vi "Mavlink Message Decode.vi"(0 "VISA in":refnum<visa-resource-name>, 1 "mav_msg":T15, 3 "error_in":errorcluster) -> (7 "VISA out":refnum<visa-resource-name>, 10 "error_out":errorcluster)   [LabVIEW 2023]
panel:
  out "AUTOPILOT_VERSION":T1
  out "VIBRATION":T2
  out "AOA_SSA":cluster{"time_usec":u64, "AOA":sgl, "SSA":sgl}
  out "AHRS3":T3
  out "AHRS":T4
  out "TERRAIN_REPORT":T5
  out "HEARTBEAT":T6
  out "POWER_STATUS":T7
  out "TIMESYNC":T8
  out "STATUSTEXT":T9(array[cluster])
  out "POSITION_TARGET_GLOBAL_INT":T10
  out "PARAM_VALUE":T11
  out "VFR_HUD":T12
  out "RC_CHANNELS":T13
  out "MISSION_CURRENT":T14
  out "NAV_CONTROLLER_OUTPUT":T16
  out "SERVO_OUTPUT_RAW":T17
  out "GLOBAL_POSITION_INT":T18
  out "ATTITUDE":T19
  out "SCALED_PRESSURE":T20
  out "RAW_IMU":T21
  out "GPS_RAW_INT":T22
  out "SYSTEM_TIME":T23
  out "SYS_STATUS":T24
  out "Message":u32[](array[numeric])
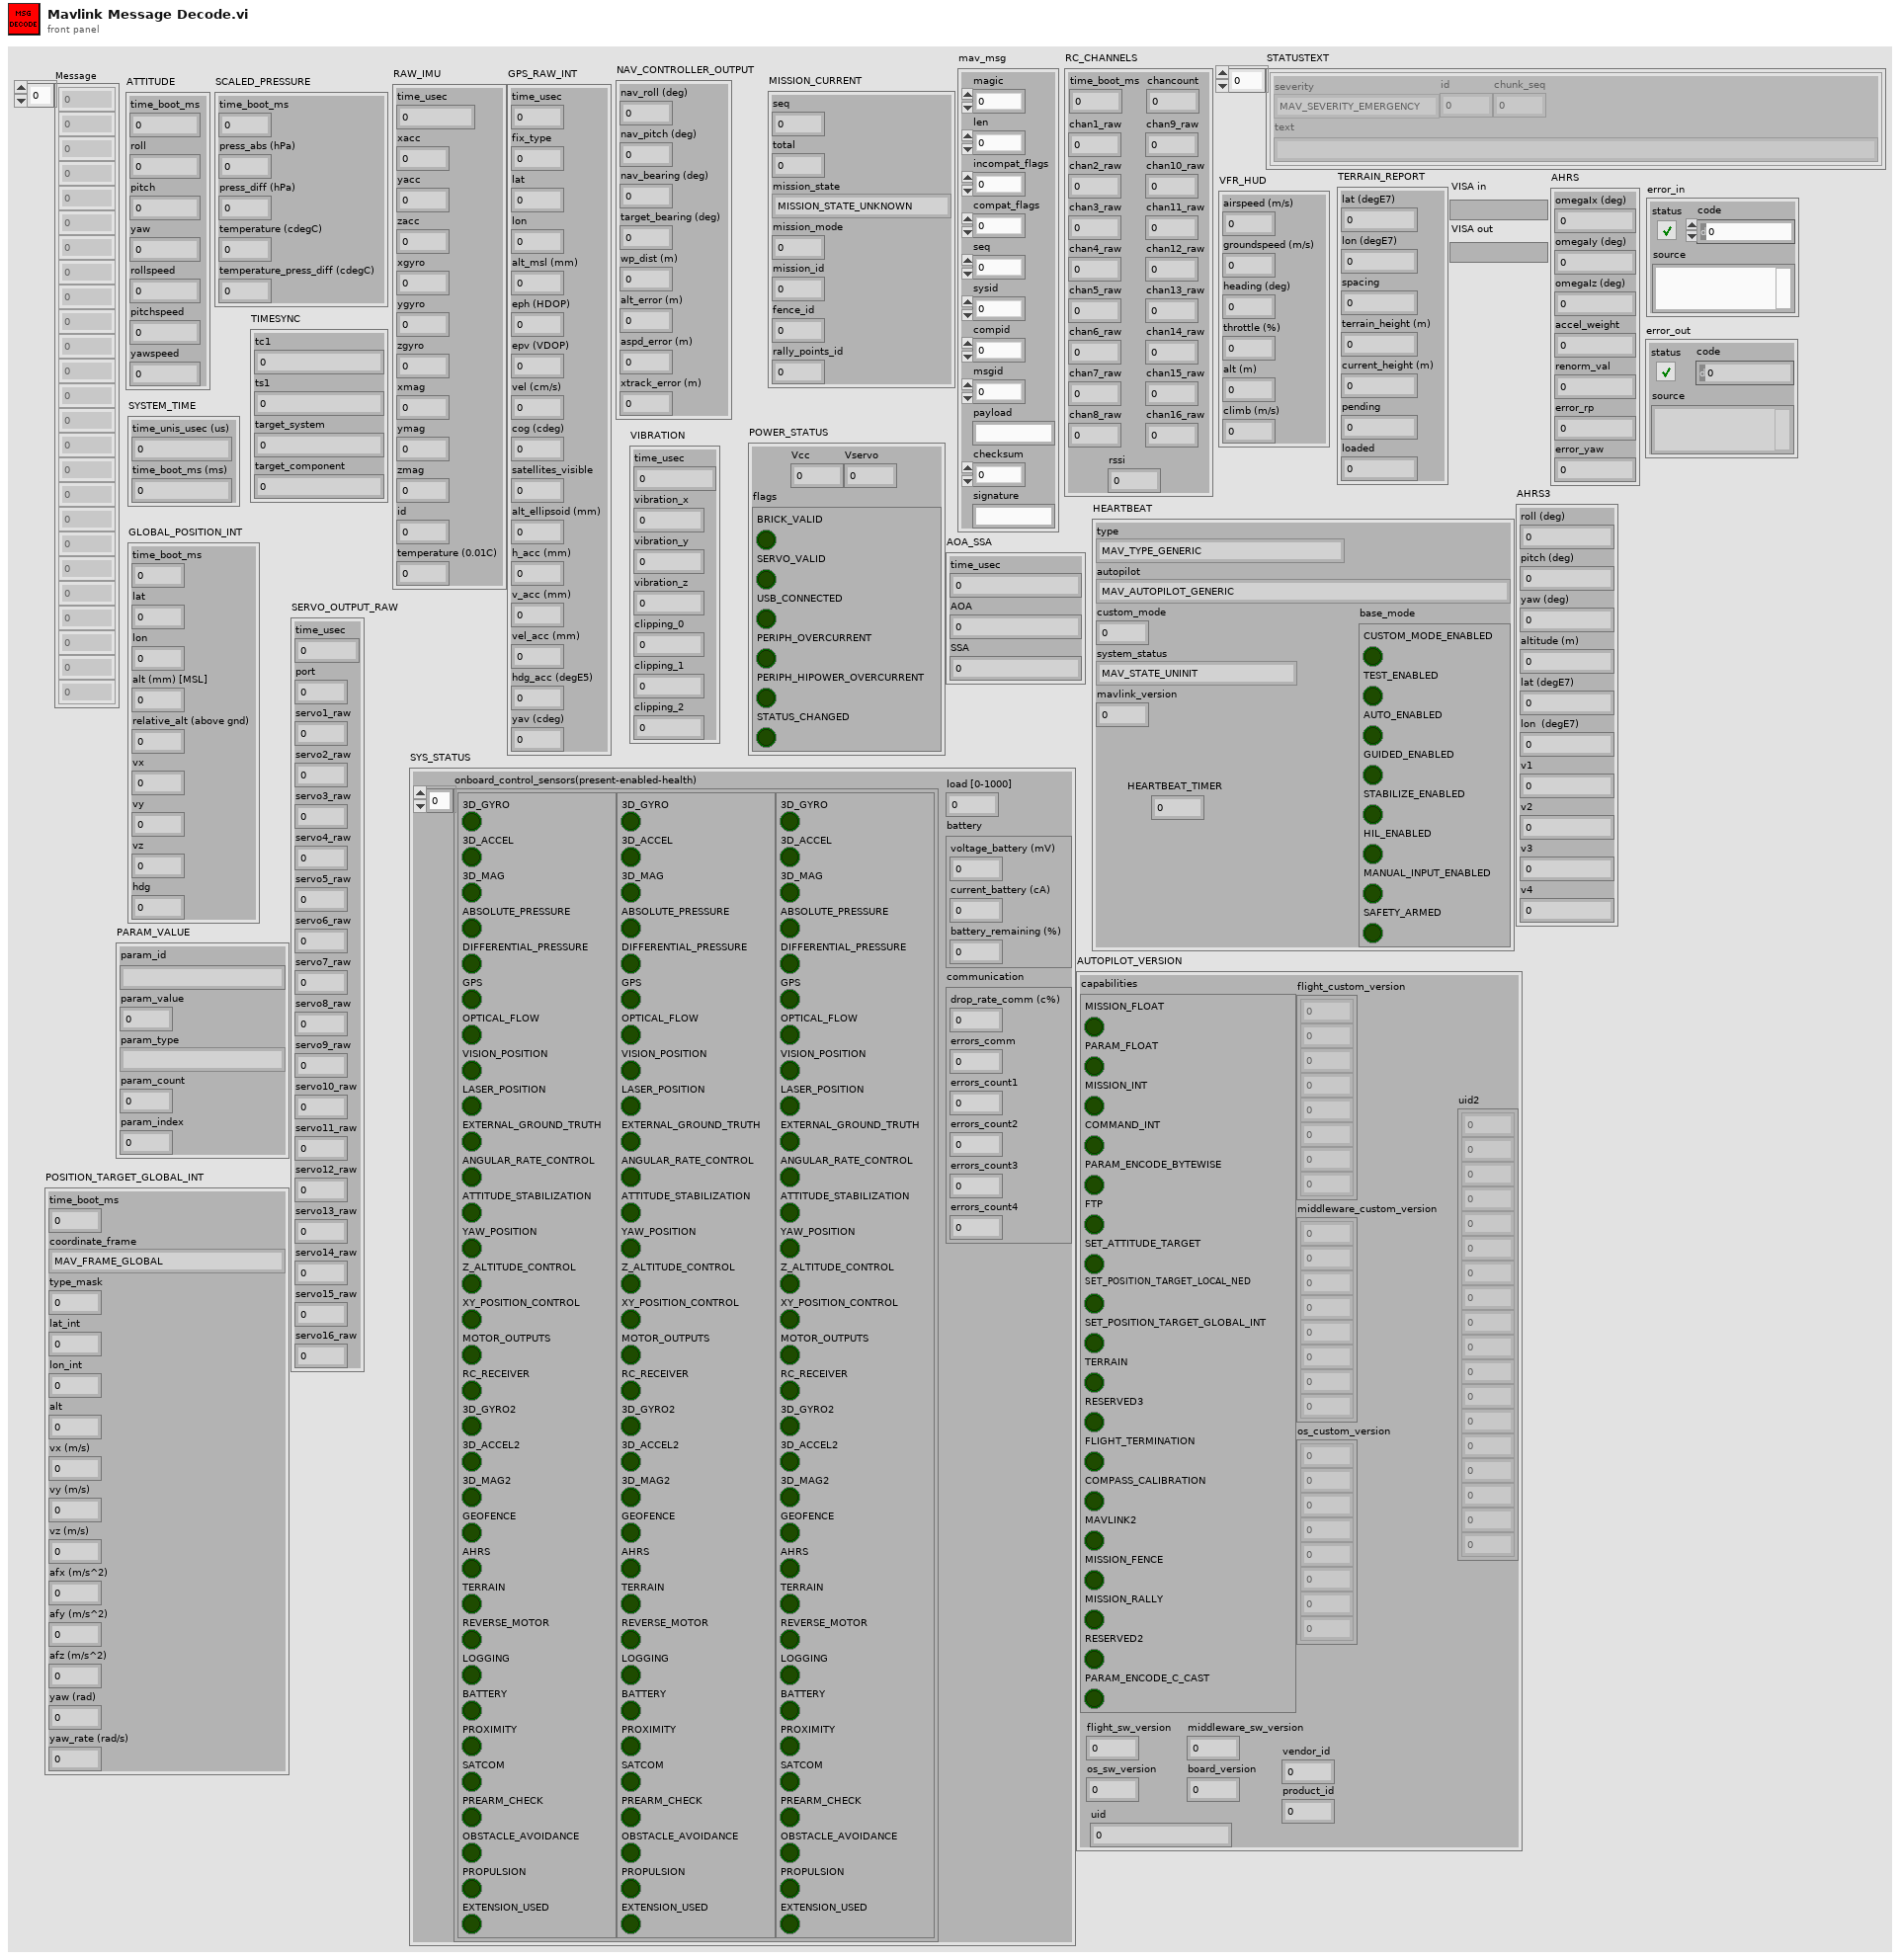
[diagram p1: front panel]
types:
  T1 = cluster{"flight_sw_version":u32, "middleware_sw_version":u32, "os_sw_version":u32, "board_version":u32, "capabilities":cluster{"MISSION_FLOAT":bool, "PARAM_FLOAT":bool, "MISSION_INT":bool, "COMMAND_INT":bool, "PARAM_ENCODE_BYTEWISE":bool, "FTP":bool, "SET_ATTITUDE_TARGET":bool, "SET_POSITION_TARGET_LOCAL_NED":bool, "SET_POSITION_TARGET_GLOBAL_INT":bool, "TERRAIN":bool, "RESERVED3":bool, "FLIGHT_TERMINATION":bool, "COMPASS_CALIBRATION":bool, "MAVLINK2":bool, "MISSION_FENCE":bool, "MISSION_RALLY":bool, "RESERVED2":bool, "PARAM_ENCODE_C_CAST":bool}, "flight_custom_version":u8[], "middleware_custom_version":u8[], "os_custom_version":u8[], "vendor_id":u16, "product_id":u16, "uid":u64, "uid2":u8[]}
  T2 = cluster{"time_usec":u64, "vibration_x":sgl, "vibration_y":sgl, "vibration_z":sgl, "clipping_0":u32, "clipping_1":u32, "clipping_2":u32}
  T3 = cluster{"roll (deg)":sgl, "pitch (deg)":sgl, "yaw (deg)":sgl, "altitude (m)":sgl, "lat (degE7)":i32, "lon  (degE7)":i32, "v1":sgl, "v2":sgl, "v3":sgl, "v4":sgl}
  T4 = cluster{"omegaIx (deg)":sgl, "omegaIy (deg)":sgl, "omegaIz (deg)":sgl, "accel_weight":sgl, "renorm_val":sgl, "error_rp":sgl, "error_yaw":sgl}
  T5 = cluster{"lat (degE7)":i32, "lon (degE7)":i32, "spacing":u16, "terrain_height (m) ":sgl, "current_height (m) ":sgl, "pending":u16, "loaded":u16}
  T6 = cluster{"type":enum8{"MAV_TYPE_GENERIC", "MAV_TYPE_FIXED_WING", "MAV_TYPE_QUADROTOR", "MAV_TYPE_COAXIAL", "MAV_TYPE_HELICOPTER", "MAV_TYPE_ANTENNA_TRACKER", "MAV_TYPE_GCS", "MAV_TYPE_AIRSHIP", "MAV_TYPE_FREE_BALLOON", "MAV_TYPE_ROCKET", "MAV_TYPE_GROUND_ROVER", "MAV_TYPE_SURFACE_BOAT", "MAV_TYPE_SUBMARINE", "MAV_TYPE_HEXAROTOR", "MAV_TYPE_OCTOROTOR", "MAV_TYPE_TRICOPTER", "MAV_TYPE_FLAPPING_WING", "MAV_TYPE_KITE", "MAV_TYPE_ONBOARD_CONTROLLER", "MAV_TYPE_VTOL_TAILSITTER_DUOROTOR", "MAV_TYPE_VTOL_TAILSITTER_QUADROTOR", "MAV_TYPE_VTOL_TILTROTOR", "MAV_TYPE_VTOL_FIXEDROTOR", "MAV_TYPE_VTOL_TAILSITTER", "MAV_TYPE_VTOL_TILTWING", "MAV_TYPE_VTOL_RESERVED5", "MAV_TYPE_GIMBAL", "MAV_TYPE_ADSB", "MAV_TYPE_PARAFOIL", "MAV_TYPE_DODECAROTOR", "MAV_TYPE_CAMERA", "MAV_TYPE_CHARGING_STATION", "MAV_TYPE_FLARM", "MAV_TYPE_SERVO", "MAV_TYPE_ODID", "MAV_TYPE_DECAROTOR", "MAV_TYPE_BATTERY", "MAV_TYPE_PARACHUTE", "MAV_TYPE_LOG", "MAV_TYPE_OSD", "MAV_TYPE_IMU", "MAV_TYPE_GPS", "MAV_TYPE_WINCH", "MAV_TYPE_GENERIC_MULTIROTOR", "MAV_TYPE_ILLUMINATOR"}, "autopilot":enum8{"MAV_AUTOPILOT_GENERIC", "MAV_AUTOPILOT_RESERVED", "MAV_AUTOPILOT_SLUGS", "MAV_AUTOPILOT_ARDUPILOTMEGA", "MAV_AUTOPILOT_OPENPILOT", "MAV_AUTOPILOT_GENERIC_WAYPOINTS_ONLY", "MAV_AUTOPILOT_GENERIC_WAYPOINTS_AND_SIMPLE_NAVIGATION_ONLY", "MAV_AUTOPILOT_GENERIC_MISSION_FULL", "MAV_AUTOPILOT_INVALID", "MAV_AUTOPILOT_PPZ", "MAV_AUTOPILOT_UDB", "MAV_AUTOPILOT_FP", "MAV_AUTOPILOT_PX4", "MAV_AUTOPILOT_SMACCMPILOT", "MAV_AUTOPILOT_AUTOQUAD", "MAV_AUTOPILOT_ARMAZILA", "MAV_AUTOPILOT_AEROB", "MAV_AUTOPILOT_ASLUAV", "MAV_AUTOPILOT_SMARTAP", "MAV_AUTOPILOT_AIRRAILS", "MAV_AUTOPILOT_REFLEX"}, "custom_mode":u32, "system_status":enum16{"MAV_STATE_UNINIT", "MAV_STATE_BOOT", "MAV_STATE_CALIBRATING", "MAV_STATE_STANDBY", "MAV_STATE_ACTIVE", "MAV_STATE_CRITICAL", "MAV_STATE_EMERGENCY", "MAV_STATE_POWEROFF", "MAV_STATE_FLIGHT_TERMINATION"}, "mavlink_version":u8, "base_mode":cluster{"CUSTOM_MODE_ENABLED":bool, "TEST_ENABLED":bool, "AUTO_ENABLED":bool, "GUIDED_ENABLED":bool, "STABILIZE_ENABLED":bool, "HIL_ENABLED":bool, "MANUAL_INPUT_ENABLED":bool, "SAFETY_ARMED":bool}, "HEARTBEAT_TIMER":u32}
  T7 = cluster{"Vcc":u16, "Vservo":u16, "flags":cluster{"BRICK_VALID":bool, "SERVO_VALID":bool, "USB_CONNECTED":bool, "PERIPH_OVERCURRENT":bool, "PERIPH_HIPOWER_OVERCURRENT":bool, "STATUS_CHANGED":bool}}
  T8 = cluster{"tc1":i64, "ts1":i64, "target_system":u8, "target_component":u8}
  T9 = cluster{"severity":enum8{"MAV_SEVERITY_EMERGENCY", "MAV_SEVERITY_ALERT", "MAV_SEVERITY_CRITICAL", "MAV_SEVERITY_ERROR", "MAV_SEVERITY_WARNING", "MAV_SEVERITY_NOTICE", "MAV_SEVERITY_INFO", "MAV_SEVERITY_DEBUG"}, "id":u16, "chunk_seq":u8, "text":string}[]
  T10 = cluster{"time_boot_ms":u32, "coordinate_frame":enum8{"MAV_FRAME_GLOBAL", "MAV_FRAME_LOCAL_NED", "MAV_FRAME_MISSION", "MAV_FRAME_GLOBAL_RELATIVE_ALT", "MAV_FRAME_LOCAL_ENU", "MAV_FRAME_GLOBAL_INT", "MAV_FRAME_GLOBAL_RELATIVE_ALT_INT", "MAV_FRAME_LOCAL_OFFSET_NED", "MAV_FRAME_BODY_NED", "MAV_FRAME_BODY_OFFSET_NED", "MAV_FRAME_GLOBAL_TERRAIN_ALT", "MAV_FRAME_GLOBAL_TERRAIN_ALT_INT", "MAV_FRAME_BODY_FRD", "MAV_FRAME_RESERVED_13", "MAV_FRAME_RESERVED_14", "MAV_FRAME_RESERVED_15", "MAV_FRAME_RESERVED_16", "MAV_FRAME_RESERVED_17", "MAV_FRAME_RESERVED_18", "MAV_FRAME_RESERVED_19", "MAV_FRAME_LOCAL_FRD", "MAV_FRAME_LOCAL_FLU"}, "type_mask":u16, "lat_int":i32, "lon_int":i32, "alt":sgl, "vx (m/s)":sgl, "vy (m/s)":sgl, "vz (m/s)":sgl, "afx (m/s^2)":sgl, "afy (m/s^2)":sgl, "afz (m/s^2)":sgl, "yaw (rad)":sgl, "yaw_rate (rad/s)":sgl}
  T11 = cluster{"param_id":string, "param_value":sgl, "param_type":enum16{"", "MAV_PARAM_TYPE_UINT8", "MAV_PARAM_TYPE_INT8", "MAV_PARAM_TYPE_UINT16", "MAV_PARAM_TYPE_INT16", "MAV_PARAM_TYPE_UINT32", "MAV_PARAM_TYPE_INT32", "MAV_PARAM_TYPE_UINT64", "MAV_PARAM_TYPE_INT64", "MAV_PARAM_TYPE_REAL32", "MAV_PARAM_TYPE_REAL64"}, "param_count":u16, "param_index":u16}
  T12 = cluster{"airspeed (m/s)":sgl, "groundspeed (m/s)":sgl, "heading (deg) ":i16, "throttle (%) ":u16, "alt (m)":sgl, "climb (m/s)":sgl}
  T13 = cluster{"time_boot_ms":u32, "chancount":u8, "chan1_raw":u16, "chan2_raw":u16, "chan3_raw":u16, "chan4_raw":u16, "chan5_raw":u16, "chan6_raw":u16, "chan7_raw":u16, "chan8_raw":u16, "chan9_raw":u16, "chan10_raw":u16, "chan11_raw":u16, "chan12_raw":u16, "chan13_raw":u16, "chan14_raw":u16, "chan15_raw":u16, "chan16_raw":u16, "rssi":u8}
  T14 = cluster{"seq":u16, "total":u16, "mission_state":enum8{"MISSION_STATE_UNKNOWN", "MISSION_STATE_NO_MISSION", "MISSION_STATE_NOT_STARTED", "MISSION_STATE_ACTIVE", "MISSION_STATE_PAUSED", "MISSION_STATE_COMPLETE"}, "mission_mode":u8, "mission_id":u32, "fence_id":u32, "rally_points_id":u32}
  T15 = cluster{"len":u8, "incompat_flags":u8, "compat_flags":u8, "seq":u8, "sysid":u8, "compid":u8, "msgid":u32, "magic":u8, "payload":string, "checksum":u16, "signature":string}
  T16 = cluster{"nav_roll (deg)":sgl, "nav_pitch (deg)":sgl, "nav_bearing (deg)":i16, "target_bearing (deg)":i16, "wp_dist (m)":u16, "alt_error (m)":sgl, "aspd_error (m)":sgl, "xtrack_error (m)":sgl}
  T17 = cluster{"time_usec":u32, "port":u8, "servo1_raw":u16, "servo2_raw":u16, "servo3_raw":u16, "servo4_raw":u16, "servo5_raw":u16, "servo6_raw":u16, "servo7_raw":u16, "servo8_raw":u16, "servo9_raw":u16, "servo10_raw":u16, "servo11_raw":u16, "servo12_raw":u16, "servo13_raw":u16, "servo14_raw":u16, "servo15_raw":u16, "servo16_raw":u16}
  T18 = cluster{"time_boot_ms":u32, "lat":i32, "lon":i32, "alt (mm) [MSL]":i32, "relative_alt (above gnd)":i32, "vx":i16, "vy":i16, "vz":i16, "hdg":u16}
  T19 = cluster{"time_boot_ms":u32, "roll":sgl, "pitch":sgl, "yaw":sgl, "rollspeed":sgl, "pitchspeed":sgl, "yawspeed":sgl}
  T20 = cluster{"time_boot_ms":u32, "press_abs (hPa)":sgl, "press_diff (hPa)":sgl, "temperature (cdegC)":i16, "temperature_press_diff (cdegC)":i16}
  T21 = cluster{"time_usec":u64, "xacc":i16, "yacc":i16, "zacc":i16, "xgyro":i16, "ygyro":i16, "zgyro":i16, "xmag":i16, "ymag":i16, "zmag":i16, "id":u8, "temperature (0.01C)":i16}
  T22 = cluster{"time_usec":u64, "fix_type":u8, "lat":i32, "lon":i32, "alt_msl (mm)":i32, "eph (HDOP)":u16, "epv (VDOP)":u16, "vel (cm/s)":u16, "cog (cdeg)":u16, "satellites_visible":u8, "alt_ellipsoid (mm)":i32, "h_acc (mm)":u32, "v_acc (mm)":u32, "vel_acc (mm)":u32, "hdg_acc (degE5)":u32, "yav (cdeg)":u16}
  T23 = cluster{"time_unis_usec (us)":u64, "time_boot_ms (ms)":u32}
  T24 = cluster{"onboard_control_sensors(present-enabled-health)":cluster{"3D_GYRO":bool, "3D_ACCEL":bool, "3D_MAG":bool, "ABSOLUTE_PRESSURE":bool, "DIFFERENTIAL_PRESSURE":bool, "GPS":bool, "OPTICAL_FLOW":bool, "VISION_POSITION":bool, "LASER_POSITION":bool, "EXTERNAL_GROUND_TRUTH":bool, "ANGULAR_RATE_CONTROL":bool, "ATTITUDE_STABILIZATION":bool, "YAW_POSITION":bool, "Z_ALTITUDE_CONTROL":bool, "XY_POSITION_CONTROL":bool, "MOTOR_OUTPUTS":bool, "RC_RECEIVER":bool, "3D_GYRO2":bool, "3D_ACCEL2":bool, "3D_MAG2":bool, "GEOFENCE":bool, "AHRS":bool, "TERRAIN":bool, "REVERSE_MOTOR":bool, "LOGGING":bool, "BATTERY":bool, "PROXIMITY":bool, "SATCOM":bool, "PREARM_CHECK":bool, "OBSTACLE_AVOIDANCE":bool, "PROPULSION":bool, "EXTENSION_USED":bool}[], "load [0-1000]":u16, "battery":cluster{"voltage_battery (mV)":u16, "current_battery (cA)":i16, "battery_remaining (%)":i8}, "communication":cluster{"drop_rate_comm (c%)":u16, "errors_comm":u16, "errors_count1":u16, "errors_count2":u16, "errors_count3":u16, "errors_count4":u16}}
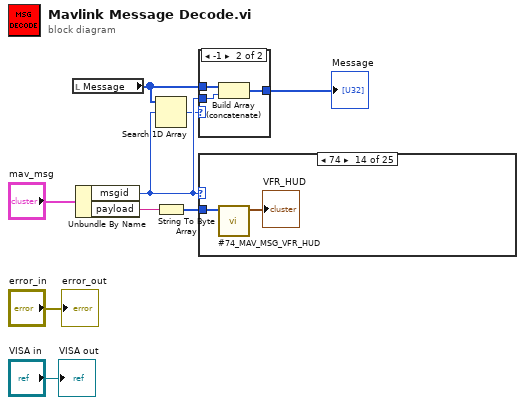
[diagram p0: block diagram]
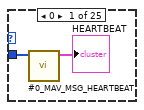
[diagram p2: hidden frame]
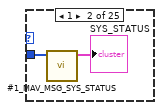
[diagram p3: hidden frame]
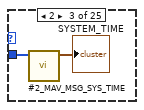
[diagram p4: hidden frame]
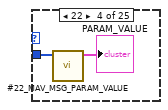
[diagram p5: hidden frame]
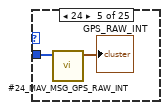
[diagram p6: hidden frame]
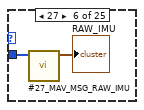
[diagram p7: hidden frame]
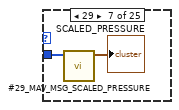
[diagram p8: hidden frame]
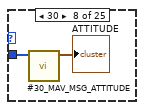
[diagram p9: hidden frame]
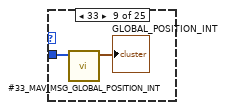
[diagram p10: hidden frame]
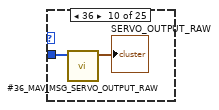
[diagram p11: hidden frame]
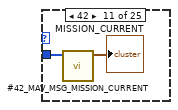
[diagram p12: hidden frame]
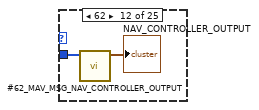
[diagram p13: hidden frame]
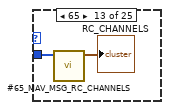
[diagram p14: hidden frame]
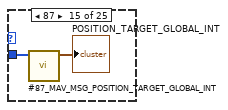
[diagram p15: hidden frame]
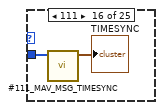
[diagram p16: hidden frame]
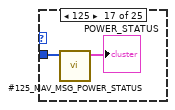
[diagram p17: hidden frame]
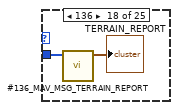
[diagram p18: hidden frame]
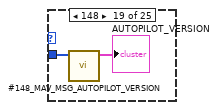
[diagram p19: hidden frame]
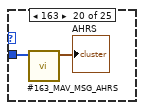
[diagram p20: hidden frame]
diagram:
  n1 = local read "Message"() -> (w3:u32[])
  n2 = Unbundle By Name("mav_msg") -> ("msgid"=w7:u32, "payload"=w8:string)
  n3 = Search 1D Array(1D array=w3, element=w7) -> (index of element=w6:i32)  [unwired: 1 in]
  n4 = String To Byte Array(string=w8) -> (unsigned byte array=w5:u8[])
  n5 = case shown="-1" w6 {
    tunnel: w3 -> [w10 w13]
    tunnel: [w10 w12] -> w4
    tunnel: w7 -> [_ w11]
    frame 1, Default {
    }
    frame -1 {
      n6 = Build Array (concatenate)(w13, w11) -> (w12:u32[])
    }
  }
  "Message" <- w4
  n7 = case shown="74" w7 {
    tunnel: w5 -> [w15 w17 w19 w21 w23 w25 w27 w29 w31 w33 w35 w37 w39 w41 w43 w45 w47 w49 w51 w53 w55 w57 w59 _ w61]
    frame 0 {
      n8 = call "#0_MAV_MSG_HEARTBEAT.vi"("mavlink_payload"=w15) -> ("HEARTBEAT"=→"HEARTBEAT":T6)  [unwired: 10 in]
    }
    frame 1 {
      n9 = call "#1_MAV_MSG_SYS_STATUS.vi"("mavlink_payload"=w17) -> ("SYS_STATUS"=→"SYS_STATUS":T24)  [unwired: 10 in]
    }
    frame 2 {
      n10 = call "#2_MAV_MSG_SYS_TIME.vi"("mavlink_payload"=w19) -> ("SYSTEM_TIME"=→"SYSTEM_TIME":T23)  [unwired: 10 in]
    }
    frame 22 {
      n11 = call "#22_MAV_MSG_PARAM_VALUE.vi"("mavlink_payload"=w21) -> ("PARAM_VALUE"=→"PARAM_VALUE":T11)  [unwired: 10 in]
    }
    frame 24 {
      n12 = call "#24_MAV_MSG_GPS_RAW_INT.vi"("mavlink_payload"=w23) -> ("GPS_RAW_INT"=→"GPS_RAW_INT":T22)  [unwired: 10 in]
    }
    frame 27 {
      n13 = call "#27_MAV_MSG_RAW_IMU.vi"("mavlink_payload"=w25) -> ("RAW_IMU"=→"RAW_IMU":T21)  [unwired: 10 in]
    }
    frame 29 {
      n14 = call "#29_MAV_MSG_SCALED_PRESSURE.vi"("mavlink_payload"=w27) -> ("SCALED_PRESSURE"=→"SCALED_PRESSURE":T20)  [unwired: 10 in]
    }
    frame 30 {
      n15 = call "#30_MAV_MSG_ATTITUDE.vi"("mavlink_payload"=w29) -> ("ATTITUDE"=→"ATTITUDE":T19)  [unwired: 10 in]
    }
    frame 33 {
      n16 = call "#33_MAV_MSG_GLOBAL_POSITION_INT.vi"("mavlink_payload"=w31) -> ("GLOBAL_POSITION_INT"=→"GLOBAL_POSITION_INT":T18)  [unwired: 10 in]
    }
    frame 36 {
      n17 = call "#36_MAV_MSG_SERVO_OUTPUT_RAW.vi"("mavlink_payload"=w33) -> ("SERVO_OUTPUT_RAW"=→"SERVO_OUTPUT_RAW":T17)  [unwired: 10 in]
    }
    frame 42 {
      n18 = call "#42_MAV_MSG_MISSION_CURRENT.vi"("mavlink_payload"=w35) -> ("MISSION_CURRENT"=→"MISSION_CURRENT":T14)  [unwired: 10 in]
    }
    frame 62 {
      n19 = call "#62_MAV_MSG_NAV_CONTROLLER_OUTPUT.vi"("mavlink_payload"=w37) -> ("NAV_CONTROLLER_OUTPUT"=→"NAV_CONTROLLER_OUTPUT":T16)  [unwired: 10 in]
    }
    frame 65 {
      n20 = call "#65_MAV_MSG_RC_CHANNELS.vi"("mavlink_payload"=w39) -> ("RC_CHANNELS"=→"RC_CHANNELS":T13)  [unwired: 10 in]
    }
    frame 74 {
      n21 = call "#74_MAV_MSG_VFR_HUD.vi"("mavlink_payload"=w41) -> ("VFR_HUD"=→"VFR_HUD":T12)  [unwired: 10 in]
    }
    frame 87 {
      n22 = call "#87_MAV_MSG_POSITION_TARGET_GLOBAL_INT.vi"("mavlink_payload"=w43) -> ("POSITION_TARGET_GLOBAL_INT"=→"POSITION_TARGET_GLOBAL_INT":T10)  [unwired: 10 in]
    }
    frame 111 {
      n23 = call "#111_MAV_MSG_TIMESYNC.vi"("mavlink_payload"=w45) -> ("TIMESYNC"=→"TIMESYNC":T8)  [unwired: 10 in]
    }
    frame 125 {
      n24 = call "#125_MAV_MSG_POWER_STATUS.vi"("mavlink_payload"=w47) -> ("POWER_STATUS"=→"POWER_STATUS":T7)  [unwired: 10 in]
    }
    frame 136 {
      n25 = call "#136_MAV_MSG_TERRAIN_REPORT.vi"("mavlink_payload"=w49) -> ("TERRAIN_REPORT"=→"TERRAIN_REPORT":T5)  [unwired: 10 in]
    }
    frame 148 {
      n26 = call "#148_MAV_MSG_AUTOPILOT_VERSION.vi"("mavlink_payload"=w51) -> ("AUTOPILOT_VERSION"=→"AUTOPILOT_VERSION":T1)  [unwired: 10 in]
    }
    frame 163 {
      n27 = call "#163_MAV_MSG_AHRS.vi"("mavlink_payload"=w53) -> ("AHRS"=→"AHRS":T4)  [unwired: 10 in]
    }
    frame 182 {
      n28 = call "#182_MAV_MSG_AHRS3.vi"("mavlink_payload"=w55) -> ("AHRS3"=→"AHRS3":T3)  [unwired: 10 in]
    }
    frame 241 {
      n29 = call "#241_MAV_MSG_VIBRATION.vi"("mavlink_payload"=w57) -> ("VIBRATION"=→"VIBRATION":T2)  [unwired: 10 in]
    }
    frame 253 {
      n30 = call "#253_MAV_MSG_STATUSTEXT.vi"("mavlink_payload"=w59) -> ("STATUSTEXT"=→"STATUSTEXT":T9)  [unwired: 10 in]
    }
    frame 255, Default {
    }
    frame 11020 {
      n31 = call "#11020_MAV_MSG_AOA_SSA.vi"("mavlink_payload"=w61) -> ("AOA_SSA"=→"AOA_SSA":cluster{"time_usec":u64, "AOA":sgl, "SSA":sgl})  [unwired: 10 in]
    }
  }
  "error_out" <- "error_in"
  "VISA out" <- "VISA in"
